vi "set_breadboard00_position.vi"(11 "UI_Data":T1={"controlTabState"=[], "pathToSTLFiles"=path "", "availableObjs"=[], "objectNames"=[], "addedObjs"=[], "selectedObj"={"Name"="", "objectFiles"=[], "center"={"X"=0.0, "Y"=0.0, "Z"=0.0}, "extent"={"X"=0.0, "Y"=0.0, "Z"=0.0}, "allowedMotion"=enum."XY", "mountOn"=enum."yArm", "Movements"=[], "extraInfo"=[], "hasPOI?"=FALSE, "POI"={"X"=0.0, "Y"=0.0, "Z"=0.0}, "posOffset"={"X"=0.0, "Y"=0.0, "Z"=0.0}, "referenceNum"=refnum}, "3DPictureObjRef"=refnum, "yPOI_0"={"X"=0.0, "Y"=0.0, "Z"=0.0}, "yPOI"={"X"=0.0, "Y"=0.0, "Z"=0.0}, "yPOI_Added?"=FALSE, "breadBoard_00"={"X"=0.0, "Y"=0.0, "Z"=0.0}, "breadBoardOriginOffset"={"X"=0.0, "Y"=0.0, "Z"=0.0}, "XYtranslateObjControls"=[], "ZtranslateObjControls"=[], "pBot_controls"=[], "pBot_VISA"="", "commandLog"="", "pBotConnected?"=FALSE, "pBot_currentEEPROMsettings"="", "realTimeInfoControls"=[], "pBot_tempSensor1"=0.0, "pBot_tempSensor2"=0.0, "realTimeInfoTextColor"=[], "disconnectPBot_Event"=refnum, "needToHomeY?"=FALSE, "pBot_relativePositioning"=FALSE, "pBot_minPos"={"X"=0.0, "Y"=0.0, "Z"=0.0}, "pBot_maxPos"={"X"=0.0, "Y"=0.0, "Z"=0.0}, "pBot_homeOffset"={"X"=0.0, "Y"=0.0, "Z"=0.0}, "textColorGreen"=9174826, "textColorRed"=16750216, "textColorGray"=9868950, "transVisualizationControls"=[], "needToHomeXY?"=FALSE, "pBot_minScanRegion"={"X"=0.0, "Y"=0.0, "Z"=0.0}, "pBot_maxScanRegion"={"X"=0.0, "Y"=0.0, "Z"=0.0}, "pBot_scanN"={"X"=0, "Y"=0, "Z"=0}, "connectedInstruments"=[], "isScanning?"=FALSE, "Wavelengths"=[], "usb2000p_controlRefs"=[], "3DPictureRef"=refnum}) -> (0 "error out":errorcluster, 3 "UI_Data out":T1={"controlTabState"=[], "pathToSTLFiles"=path "", "availableObjs"=[], "objectNames"=[], "addedObjs"=[], "selectedObj"={"Name"="", "objectFiles"=[], "center"={"X"=0.0, "Y"=0.0, "Z"=0.0}, "extent"={"X"=0.0, "Y"=0.0, "Z"=0.0}, "allowedMotion"=enum."XY", "mountOn"=enum."yArm", "Movements"=[], "extraInfo"=[], "hasPOI?"=FALSE, "POI"={"X"=0.0, "Y"=0.0, "Z"=0.0}, "posOffset"={"X"=0.0, "Y"=0.0, "Z"=0.0}, "referenceNum"=refnum}, "3DPictureObjRef"=refnum, "yPOI_0"={"X"=0.0, "Y"=0.0, "Z"=0.0}, "yPOI"={"X"=0.0, "Y"=0.0, "Z"=0.0}, "yPOI_Added?"=FALSE, "breadBoard_00"={"X"=0.0, "Y"=0.0, "Z"=0.0}, "breadBoardOriginOffset"={"X"=0.0, "Y"=0.0, "Z"=0.0}, "XYtranslateObjControls"=[], "ZtranslateObjControls"=[], "pBot_controls"=[], "pBot_VISA"="", "commandLog"="", "pBotConnected?"=FALSE, "pBot_currentEEPROMsettings"="", "realTimeInfoControls"=[], "pBot_tempSensor1"=0.0, "pBot_tempSensor2"=0.0, "realTimeInfoTextColor"=[], "disconnectPBot_Event"=refnum, "needToHomeY?"=FALSE, "pBot_relativePositioning"=FALSE, "pBot_minPos"={"X"=0.0, "Y"=0.0, "Z"=0.0}, "pBot_maxPos"={"X"=0.0, "Y"=0.0, "Z"=0.0}, "pBot_homeOffset"={"X"=0.0, "Y"=0.0, "Z"=0.0}, "textColorGreen"=9174826, "textColorRed"=16750216, "textColorGray"=9868950, "transVisualizationControls"=[], "needToHomeXY?"=FALSE, "pBot_minScanRegion"={"X"=0.0, "Y"=0.0, "Z"=0.0}, "pBot_maxScanRegion"={"X"=0.0, "Y"=0.0, "Z"=0.0}, "pBot_scanN"={"X"=0, "Y"=0, "Z"=0}, "connectedInstruments"=[], "isScanning?"=FALSE, "Wavelengths"=[], "usb2000p_controlRefs"=[], "3DPictureRef"=refnum})   [LabVIEW 2015]
uses:
  controls/UI Data.ctl
  processedObjectInfo.ctl
  controls/scanInstrumentInfo.ctl
  <vilib>/picture/3D Picture Control/NI_3D Picture Control.lvlib
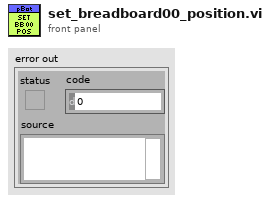
[diagram p1: front panel]
types:
  T1 = typedef "UI Data.ctl" = cluster{"controlTabState":bool[], "pathToSTLFiles":path, "availableObjs":T2[], "objectNames":string[], "addedObjs":T2[], "selectedObj":T2, "3DPictureObjRef":refnum<vi>, "yPOI_0":cluster{"X":dbl, "Y":dbl, "Z":dbl}, "yPOI":cluster{"X":dbl, "Y":dbl, "Z":dbl}, "yPOI_Added?":bool, "breadBoard_00":cluster{"X":dbl, "Y":dbl, "Z":dbl}, "breadBoardOriginOffset":cluster{"X":dbl, "Y":dbl, "Z":dbl}, "XYtranslateObjControls":refnum<vi>[], "ZtranslateObjControls":refnum<vi>[], "pBot_controls":refnum<vi>[], "pBot_VISA":refnum<visa-resource-name>, "commandLog":string, "pBotConnected?":bool, "pBot_currentEEPROMsettings":string, "realTimeInfoControls":refnum<vi>[], "pBot_tempSensor1":dbl, "pBot_tempSensor2":dbl, "realTimeInfoTextColor":u32[], "disconnectPBot_Event":refnum<user-event>, "needToHomeY?":bool, "pBot_relativePositioning":bool, "pBot_minPos":cluster{"X":dbl, "Y":dbl, "Z":dbl}, "pBot_maxPos":cluster{"X":dbl, "Y":dbl, "Z":dbl}, "pBot_homeOffset":cluster{"X":dbl, "Y":dbl, "Z":dbl}, "textColorGreen":u32, "textColorRed":u32, "textColorGray":u32, "transVisualizationControls":refnum<vi>[], "needToHomeXY?":bool, "pBot_minScanRegion":cluster{"X":sgl, "Y":sgl, "Z":sgl}, "pBot_maxScanRegion":cluster{"X":sgl, "Y":sgl, "Z":sgl}, "pBot_scanN":cluster{"X":u16, "Y":u16, "Z":u16}, "connectedInstruments":T3[], "isScanning?":bool, "Wavelengths":dbl[], "usb2000p_controlRefs":refnum<vi>[], "3DPictureRef":refnum<vi>}
  T2 = typedef "processedObjectInfo.ctl" = cluster{"Name":string, "objectFiles":cluster{"Location":path, "Color":cluster{"R":dbl, "G":dbl, "B":dbl, "A":dbl}}[], "center":cluster{"X":dbl, "Y":dbl, "Z":dbl}, "extent":cluster{"X":dbl, "Y":dbl, "Z":dbl}, "allowedMotion":enum16{"XY", "Z"}, "mountOn":enum16{"yArm", "breadBoard"}, "Movements":cluster{"Type":enum16{"rr", "ra", "tr", "ta"}, "vector":cluster{"X":dbl, "Y":dbl, "Z":dbl}, "scalar":dbl}[], "extraInfo":cluster{"parameter":string, "dataType":string, "vector":cluster{"X":dbl, "Y":dbl, "Z":dbl}, "scalar":dbl}[], "hasPOI?":bool, "POI":cluster{"X":dbl, "Y":dbl, "Z":dbl}, "posOffset":cluster{"X":dbl, "Y":dbl, "Z":dbl}, "referenceNum":refnum<vi>}
  T3 = typedef "scanInstrumentInfo.ctl" = cluster{"Name":string, "VISAname":refnum<visa-resource-name>, "1D_dataArraySize":u16, "extraInfo":variant, "error":errorcluster}
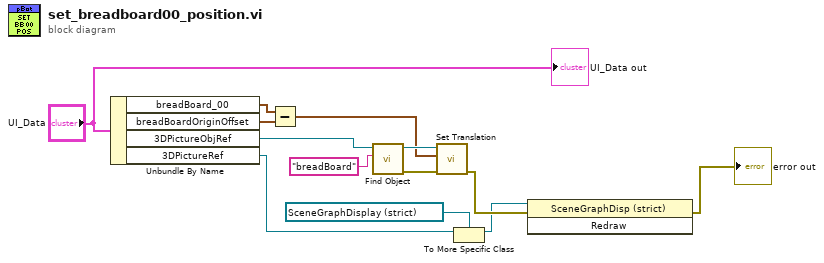
[diagram p0: block diagram]
diagram:
  n1 = Unbundle By Name("UI_Data") -> ("breadBoard_00"=w6:cluster{"X":dbl, "Y":dbl, "Z":dbl}, "breadBoardOriginOffset"=w11:cluster{"X":dbl, "Y":dbl, "Z":dbl}, "3DPictureObjRef"=w7:refnum<vi>, "3DPictureRef"=w3:refnum<vi>)
  n2 = Subtract(x=w6, y=w11) -> (x-y=w8:cluster{"X":dbl, "Y":dbl, "Z":dbl})
  n3 = call <vilib>:"Find Object.vi"("Object Name"="breadBoard", "Scene Refnum"=w7) -> ("error out"=w10:errorcluster, "Object Refnum"=w12:refnum<vi>)  [unwired: 8 in]
  n4 = call <vilib>:"Set Translation.vi"("error in (no error)"=w10, "Translation"=w8, "Scene Object"=w12) -> ("error out"=w5:errorcluster)  [unwired: 7 in, 1 out]
  n5 = To More Specific Class(target class=refnum<vi> refnum ("3D Picture"), reference=w3) -> (specific class reference=w2:refnum<vi>)  [unwired: 1 in, 1 out]
  n6 = invoke class="SceneGraphDisp (strict)" method="Redraw"(reference=w2, error in=w5) -> (error out=→"error out":errorcluster)  [unwired: 1 in, 2 out]
  "UI_Data out" <- "UI_Data"
